vi "Main.vi"(11 "Module Admin":refnum<class "Delacor_lib_QMH_Module Admin.lvclass">) -> ()   [LabVIEW 2020, in "Contabilidad.lvlib"]
doc: "This template is based off of the Queued Message Handler design pattern and the Queued Message Handler project template that ships with LabVIEW.\n\nThe main difference is that the queue is private to this module and communication between modules is performed via Broadcast and Request events.\n\nRequest events are wrapped in public API methods and are handled in the Event Handling Loop (EHL) of this VI. Any module can register for Broadcast events sent by this module. The EHL generates messages based on user interface actions.\n\nThe Message Handling Loop (MHL) processes messages generated by the EHL, or by other messages. The messages are string values, so new messages can be added easily to the Message Cases case structure in the MHL. Each message cluster can also provide an optional value for Message Data, which is a variant that can be converted to whatever message-specific data is required.\n_____\nBased on DQMH Project Template 6.0.0.91."
uses:
  Contabilidad.lvlib
  <vilib>/Delacor/Delacor QMH/Libraries/Module Admin_class/Delacor_lib_QMH_Module Admin.lvclass
  Module Data--cluster.ctl
  Stop Argument--cluster.ctl
  <vilib>/Delacor/Delacor QMH/Libraries/Message Queue_class/Delacor_lib_QMH_Message Queue.lvclass/Delacor_lib_QMH_Message Queue.ctl
  <vilib>/Delacor/Delacor QMH/Libraries/Module Admin_class/Delacor_lib_QMH_Module Admin.lvclass/Delacor_lib_QMH_Module Admin.ctl
  <vilib>/Utility/miscctls.llb/LVPointTypeDef.ctl
  <vilib>/Delacor/Delacor QMH/Libraries/Message Queue_class/Delacor_lib_QMH_Enqueue Message (Single).vi
  <vilib>/Delacor/Delacor QMH/Libraries/Module Admin_class/Delacor_lib_QMH_Get External Launch.vi
  <vilib>/Utility/error.llb/Error Cluster From Error Code.vi
  <vilib>/ErrorRing/Error Ring.xnode
  <vilib>/Delacor/Delacor QMH/Libraries/Message Queue_class/Delacor_lib_QMH_Message Queue.lvclass
  Paquetes Disponibles/Paquetes Disponibles.lvlib
panel:
  out "error out":errorcluster
  out "Status":string
types:
  T1 = typedef "Contabilidad.lvlib/Request Events--cluster.ctl" = cluster{"Stop Module":refnum<user-event>, "Show Panel":refnum<user-event>, "Hide Panel":refnum<user-event>, "Get Module Execution Status":refnum<user-event>, "Show Diagram":refnum<user-event>}
  T2 = typedef "Paquetes Disponibles.lvlib/Broadcast Events--cluster.ctl" = cluster{"Module Did Init":refnum<user-event>, "Status Updated":refnum<user-event>, "Error Reported":refnum<user-event>, "Module Did Stop":refnum<user-event>, "Update Module Execution Status":refnum<user-event>, "Servicio Seleccionado":refnum<user-event>, "Actualizar Credito":refnum<user-event>, "Actualizar Cambio":refnum<user-event>}
  T3 = typedef "Contabilidad.lvlib/Module Data--cluster.ctl" = cluster{"Status":string}
  T4 = enum32{"invalid lock state", "Not Locked", "Locked (No Password)", "Password-protected"}
  T5 = typedef "Contabilidad.lvlib/Stop Argument--cluster.ctl" = cluster{"Origin":string, "Exit via Stop Module Req?":bool, "Wait for Module to stop?":bool}
  T6 = typedef "LVPointTypeDef.ctl" = cluster{"Horizontal":i16, "Vertical":i16}
  T7 = enum32{"Invalid", "Standard", "Closed", "Hidden", "Minimized", "Maximized"}
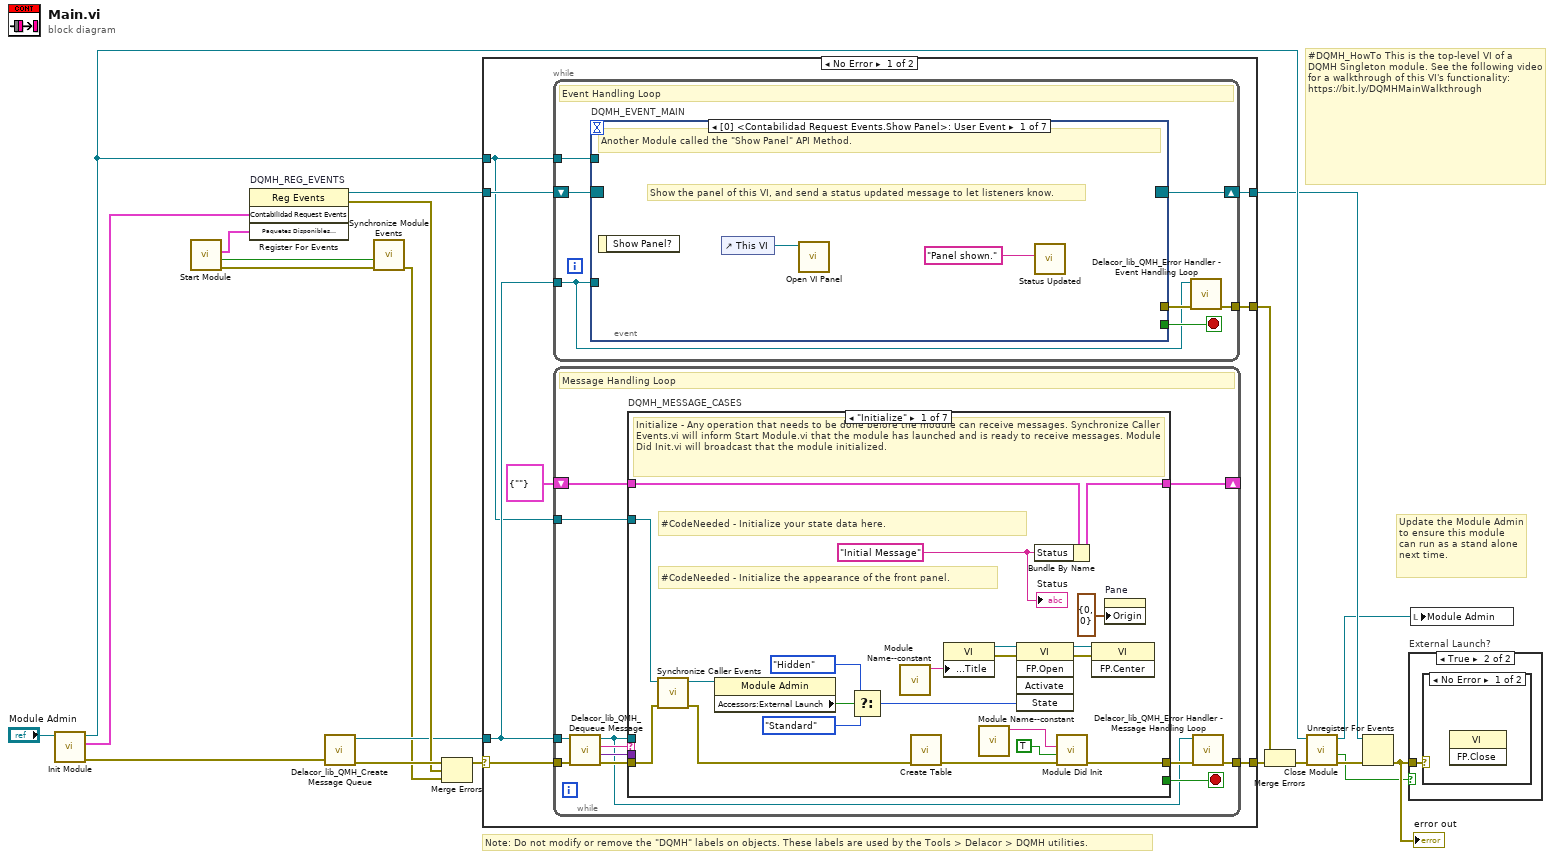
[diagram p0: block diagram]
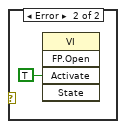
[diagram p3: hidden frame]
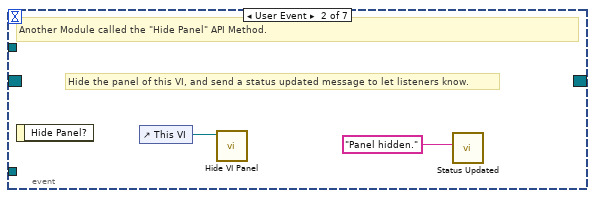
[diagram p4: hidden frame]
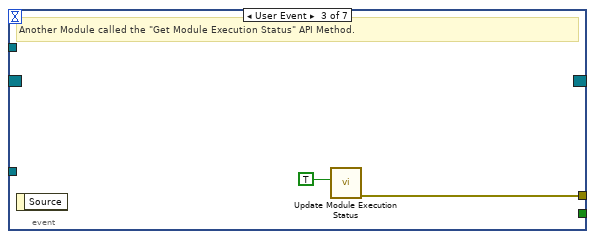
[diagram p5: hidden frame]
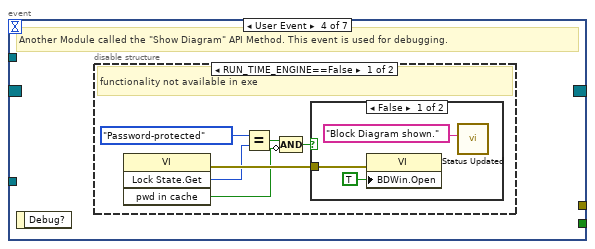
[diagram p6: hidden frame]
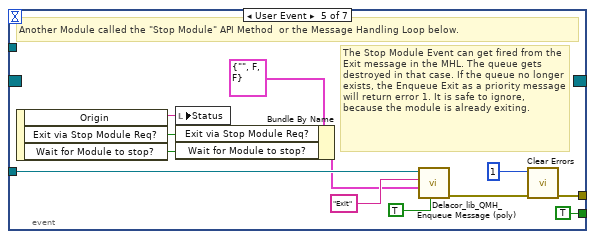
[diagram p9: hidden frame]
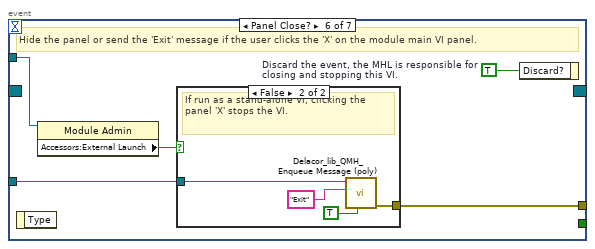
[diagram p10: hidden frame]
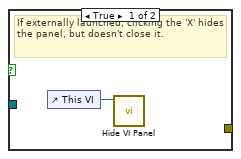
[diagram p11: hidden frame]
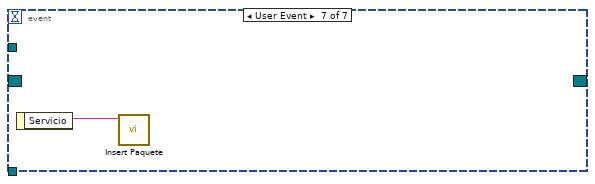
[diagram p12: hidden frame]
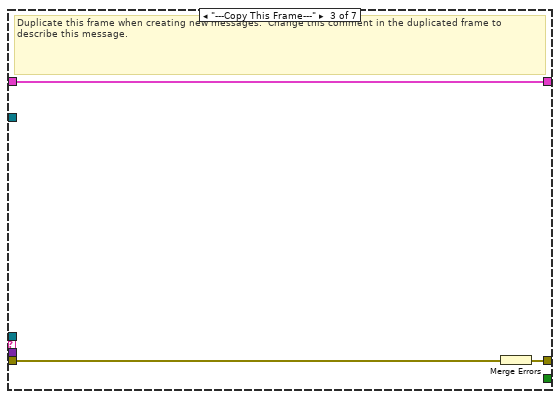
[diagram p14: hidden frame]
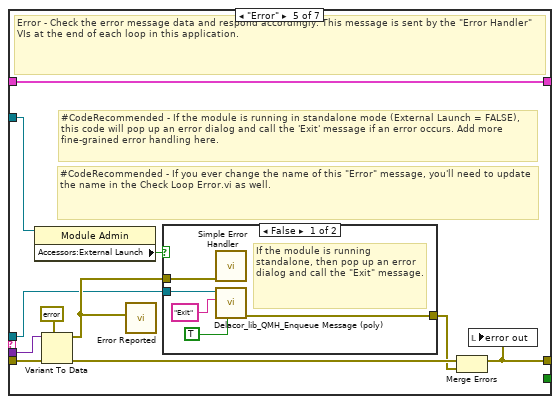
[diagram p16: hidden frame]
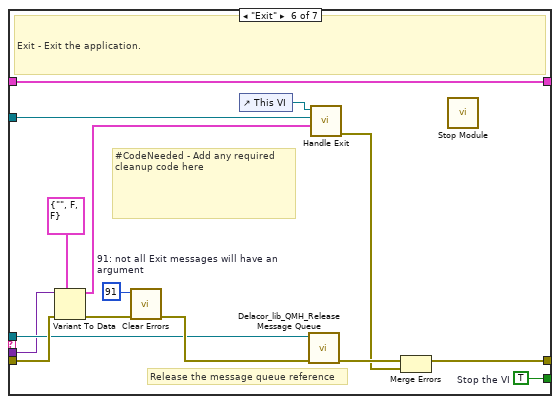
[diagram p18: hidden frame]
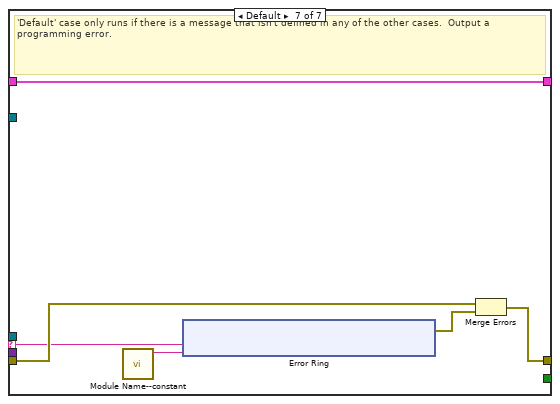
[diagram p19: hidden frame]
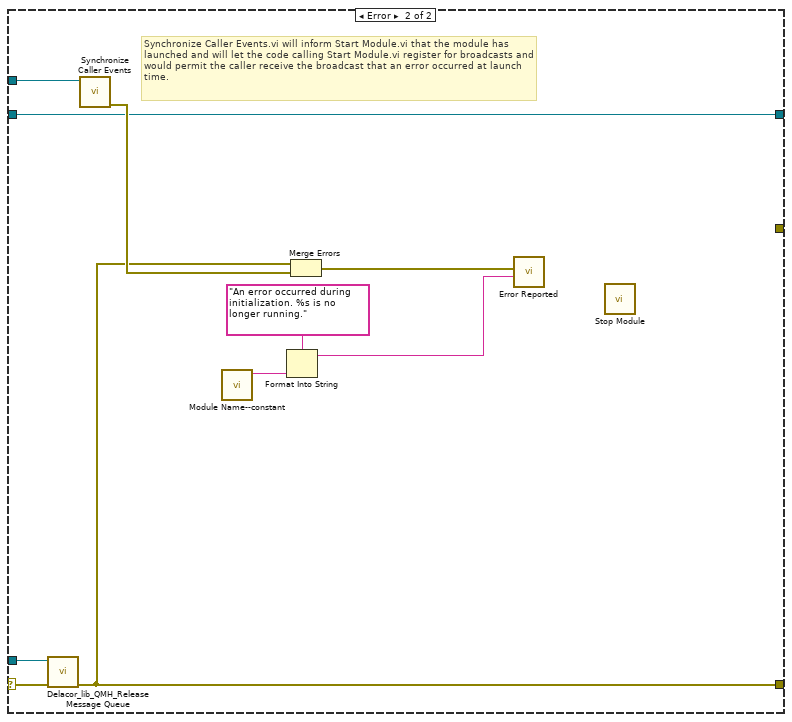
[diagram p20: hidden frame]
diagram:
  # "#DQMH_HowTo This is the top-level VI of a DQMH Singleton module. See the following video for a walkthrough of this VI's functionality: https://bit.ly/DQMHMainWalkthrough"
  # "Note: Do not modify or remove the \"DQMH\" labels on objects. These labels are used by the Tools > Delacor > DQMH utilities."
  # "Update the Module Admin to ensure this module can run as a stand alone next time."
  n1 = call "Init Module.vi"("Singleton Module Admin in"="Module Admin") -> ("error out"=w20:errorcluster, "Contabilidad Request Events"=w9:T1, "Singleton Module Admin out"=w12:refnum<class "Delacor_lib_QMH_Module Admin.lvclass">)  [unwired: 8 in]
  n2 = call "Start Module.vi"() -> ("error out"=w1:errorcluster, "Wait for Event Sync?"=w3:bool, "Paquetes Disponibles Broadcast Events"=w4:T2)  [unwired: 8 in, 1 out]
  n3 = register-events "DQMH_REG_EVENTS"(w9, w4) -> (reference out=w10:refnum<event-registration>, error out=w13:errorcluster)  [unwired: 2 in]
  n4 = call <vilib>:"Delacor_lib_QMH_Create Message Queue.vi"("error in"=w20) -> ("error out"=w15:errorcluster, "Message Queue"=w8:refnum<class "Delacor_lib_QMH_Message Queue.lvclass">)  [unwired: 9 in]
  n5 = call "Synchronize Module Events.vi"("error in"=w1, "Wait for Event Sync?"=w3) -> ("error out"=w2:errorcluster)  [unwired: 9 in]
  n6 = Merge Errors(w15, w13, w2) -> (w14:errorcluster)
  n7 = case shown="No Error" w14 {
    selector: w14 -> [w27 w162]
    tunnel: [w29 w161] -> w21
    tunnel: [w26 w167] -> w11
    tunnel: w10 -> [w24 w167]
    tunnel: w8 -> [w23 w160]
    tunnel: [w28 _] -> w18
    tunnel: w12 -> [w22 w163]
    frame No Error {
      n8 = while {
        tunnel: w23 -> [w30]
        shift-right: [w33] -> w26
        shift-left: w24 -> [w34]
        tunnel: [w35] -> w28
        tunnel: w22 -> [w31]
        stop <- w32 stop-if-true
        # "Event Handling Loop"
        n9 = event "DQMH_EVENT_MAIN" shown="[0] <Contabilidad Request Events.Show Panel>: User Event" {
          selector: w34 -> [_ _ _ _ _ _ _]
          dyn-events: [_ _ _ _ _ _ _] -> w33
          timeout: _ -> [_ _ _ _ _ _ _]
          tunnel: [_ _ _ _ TRUE ("Discard?") _ _] -> w32
          tunnel: w30 -> [_ _ _ _ w59 w66 _]
          tunnel: [_ _ w42 _ w62 w68 _] -> w36
          tunnel: w31 -> [_ _ _ _ _ w65 _]
          event User Event {
            # "Show the panel of this VI, and send a status updated message to let listeners know."
            # "Another Module called the \"Show Panel\" API Method."
            n10 = event-data() -> ()  [unwired: 1 in, 1 out]
            n11 = control-ref of="This VI"() -> (w38:refnum<vi>)
            n12 = call "Open VI Panel.vi"("VI"=w38) -> ()  [unwired: 10 in, 1 out]
            n13 = call "Status Updated.vi"("Status"="Panel shown." ("format string")) -> ()  [unwired: 10 in, 1 out]
          }
          event User Event {
            # "Hide the panel of this VI, and send a status updated message to let listeners know."
            # "Another Module called the \"Hide Panel\" API Method."
            n14 = event-data() -> ()  [unwired: 1 in, 1 out]
            n15 = control-ref of="This VI"() -> (w40:refnum<vi>)
            n16 = call "Hide VI Panel.vi"("VI"=w40) -> ()  [unwired: 10 in, 1 out]
            n17 = call "Status Updated.vi"("Status"="Panel hidden." ("format string")) -> ()  [unwired: 10 in, 1 out]
          }
          event User Event {
            # "Another Module called the \"Get Module Execution Status\" API Method."
            n18 = event-data() -> ()  [unwired: 1 in, 1 out]
            n19 = call "Update Module Execution Status.vi"("Running?"=TRUE) -> ("error out"=w42:errorcluster)  [unwired: 10 in]
          }
          event User Event {
            # "Another Module called the \"Show Diagram\" API Method. This event is used for debugging."
            n20 = event-data() -> ()  [unwired: 1 in, 1 out]
            n21 = disable-structure shown="RUN_TIME_ENGINE==False" {
              frame condition #0 (active) {
                # "functionality not available in exe"
                n22 = invoke class="VI" method="Lock State.Get"() -> (error out=w48:errorcluster, "Get Lock State"=w47:T4, "pwd in cache"=w44:bool)  [unwired: 4 in, 1 out]
                n23 = Equal?(x=T4."Password-protected", y=w47) -> (x = y?=w45:bool)
                n24 = Compound Arithmetic op=AND(w45, invert w44) -> (w43:bool)
                n25 = case shown="False" w43 {
                  tunnel: w48 -> [w51 _]
                  frame False {
                    n26 = property class="VI"(error in=w51, "BDWin.Open"=TRUE ("Block Diagram Window:Open")) -> ()  [unwired: 1 in, 2 out]
                    n27 = call "Status Updated.vi"("Status"="Block Diagram shown." ("format string")) -> ()  [unwired: 10 in, 1 out]
                  }
                  frame True {
                    # "Password-protected VI, and the password is not in the cache. Do not show the diagram."
                  }
                }
              }
              frame condition #1 {
              }
            }
          }
          event User Event {
            # "The Stop Module Event can get fired from the Exit message in the MHL. The queue gets destroyed in that case. If the queue no longer exists, the Enqueue Exit as a priority message will return error 1. It is safe to ignore, because the module is already exiting."
            # "Another Module called the \"Stop Module\" API Method  or the Message Handling Loop below."
            n28 = event-data() -> ("Origin"=w58:string, "Exit via Stop Module Req?"=w54:bool, "Wait for Module to stop?"=w53:bool)  [unwired: 1 in]
            n29 = local write "Status"(w58) -> ()
            n30 = Bundle By Name(cluster=T5 {"Origin"="", "Exit via Stop Module Req?"=FALSE, "Wait for Module to stop?"=FALSE} ("Stop Argument"), "Exit via Stop Module Req?"=w54, "Wait for Module to stop?"=w53) -> (w52:T5)
            n31 = call-poly <vilib>:"Delacor_lib_QMH_Enqueue Message (poly).vi"("Priority Message? (F)"=TRUE, "Message Data"=w52, "Message"="Exit", "Message Queue in"=w59) -> ("error out"=w63:errorcluster)  [unwired: 6 in, 1 out]
            n32 = call <vilib>:"Clear Errors.vi"("error in (no error)"=w63, "specific error code to clear (0: all)"=1) -> ("error out"=w62:errorcluster)  [unwired: 4 in, 1 out]
          }
          event Panel Close? {
            w67 = TRUE  # Discard the event, the MHL is responsible for closing and stopping this VI.
            # "Hide the panel or send the 'Exit' message if the user clicks the 'X' on the module main VI panel."
            n33 = event-data() -> ()  [unwired: 1 in, 1 out]
            n34 = property class="Module Admin"(reference=w65) -> ("Accessors:External Launch"=w64:bool)  [unwired: 1 in, 2 out]
            n35 = case shown="False" w64 {
              tunnel: w66 -> [_ w72]
              tunnel: [_ w73] -> w68
              frame True {
                # "If externally launched, clicking the 'X' hides the panel, but doesn't close it."
                n36 = control-ref of="This VI"() -> (w69:refnum<vi>)
                n37 = call "Hide VI Panel.vi"("VI"=w69) -> ()  [unwired: 10 in, 1 out]
              }
              frame False {
                # "If run as a stand-alone VI, clicking the panel 'X' stops the VI."
                n38 = call-poly <vilib>:"Delacor_lib_QMH_Enqueue Message (poly).vi"("Priority Message? (F)"=TRUE, "Message"="Exit", "Message Queue in"=w72) -> ("error out"=w73:errorcluster)  [unwired: 7 in, 1 out]
              }
            }
            n39 = event-data("Discard?"=w67) -> ()  [unwired: 1 in, 1 out]
          }
          event User Event {
            n40 = event-data() -> ("Servicio"=w74:string)  [unwired: 1 in]
            n41 = call "Insert Paquete.vi"("Paquete"=w74) -> ()  [unwired: 10 in, 1 out]
          }
        }
        n42 = call-dynamic "Delacor_lib_QMH_Error Handler - Event Handling Loop.vi"("error in"=w36, "Message Queue in"=w30) -> ("dup error in"=w35:errorcluster)  [unwired: 8 in, 1 out]
      }
      n43 = while {
        tunnel: w23 -> [w77]
        shift-right: [w81] -> _
        shift-left: T3 {"Status"=""} ("Data Cluster") -> [w82]
        tunnel: w27 -> [w85]
        tunnel: [w83] -> w29
        tunnel: w22 -> [w75]
        stop <- w80 stop-if-true
        # "Message Handling Loop"
        n44 = call-dynamic "Delacor_lib_QMH_Dequeue Message.vi"("error in"=w85, "Message Queue in"=w77) -> ("error out"=w84:errorcluster, "Message Data"=w78:variant, "Message"=w79:string, "Message Queue out"=w76:refnum<class "Delacor_lib_QMH_Message Queue.lvclass">)  [unwired: 6 in]
        n45 = case "DQMH_MESSAGE_CASES" shown="\"Initialize\"" w79 {
          selector: w79 -> [_ _ _ _ _ _ w147]
          tunnel: w76 -> [_ _ _ _ w117 w139 _]
          tunnel: w84 -> [w105 w109 w112 w114 w124 w145 w149]
          tunnel: [w104 w109 w111 w114 w120 w142 w150] -> w86
          tunnel: w82 -> [w95 w108 w110 w113 w119 w138 w148]
          tunnel: [w94 w108 w110 w113 w119 w138 w148] -> w81
          tunnel: [_ _ _ _ _ w137 _] -> w80
          tunnel: w78 -> [_ _ _ _ w118 w136 _]
          tunnel: w75 -> [w96 _ _ _ w116 w131 _]
          frame "Initialize" {
            w90 = "Initial Message" ("Initial Message")
            # "#CodeNeeded - Initialize the appearance of the front panel."
            # "#CodeNeeded - Initialize your state data here."
            # "Initialize - Any operation that needs to be done before the module can receive messages. Synchronize Caller Events.vi will inform Start Module.vi that the module has launched and is ready to receive messages. Module Did Init.vi will broadcast that the module initialized."
            n46 = call "Synchronize Caller Events.vi"("error in (no error)"=w105, "Singleton Module Admin in"=w96) -> ("error out"=w87:errorcluster, "Singleton Module Admin out"=w91:refnum<class "Delacor_lib_QMH_Module Admin.lvclass">)  [unwired: 8 in]
            n47 = property class="Module Admin"(reference=w91) -> ("Accessors:External Launch"=w100:bool)  [unwired: 1 in, 2 out]
            n48 = Select(t=T7."Hidden" ("State"), s=w100, f=T7."Standard" ("State")) -> (s? t:f=w97:T7)
            n49 = call "Module Name--constant.vi"() -> ("Module Name"=w103:string)  [unwired: 11 in]
            n50 = call "Create Table.vi"("error in (no error)"=w87) -> ("error out"=w88:errorcluster)  [unwired: 10 in]
            n51 = property class="VI"("Front Panel.Title"=w103) -> (reference out=w102:refnum<vi>, error out=w107:errorcluster)  [unwired: 2 in]
            n52 = call "Module Name--constant.vi"() -> ("Module Name"=w92:string)  [unwired: 11 in]
            n53 = invoke class="VI" method="FP.Open"(reference=w102, error in=w107, "State"=w97) -> (reference out=w101:refnum<vi>, error out=w106:errorcluster)  [unwired: 2 in, 3 out]
            n54 = Bundle By Name(cluster=w95, "Status"=w90) -> (w94:T3)
            n55 = call "Module Did Init.vi"("error in (no error)"=w88, "Initialized?"=TRUE, "Origin"=w92) -> ("error out"=w104:errorcluster)  [unwired: 8 in]
            n56 = invoke class="VI" method="FP.Center"(reference=w101, error in=w106) -> ()  [unwired: 1 in, 3 out]
            n57 = property on="Pane" class="Pane"("Origin"=T6 {"Horizontal"=0, "Vertical"=0}) -> ()  [unwired: 2 in, 2 out]
            "Status" <- w90
          }
          frame "---Module Specific---" {
            # "Separator -- The following cases handle messages specific to this Module."
          }
          frame "---Copy This Frame---" {
            # "Duplicate this frame when creating new messages.  Change this comment in the duplicated frame to describe this message."
            n58 = Merge Errors(w112) -> (w111:errorcluster)
          }
          frame "---Exit and Error Handling---" {
            # "Separator - The following cases handle errors and exit messages."
          }
          frame "Error" {
            # "#CodeRecommended - If you ever change the name of this \"Error\" message, you'll need to update the name in the Check Loop Error.vi as well."
            # "#CodeRecommended - If the module is running in standalone mode (External Launch = FALSE), this code will pop up an error dialog and call the 'Exit' message if an error occurs. Add more fine-grained error handling here."
            # "Error - Check the error message data and respond accordingly. This message is sent by the \"Error Handler\" VIs at the end of each loop in this application."
            n59 = property class="Module Admin"(reference=w116) -> ("Accessors:External Launch"=w115:bool)  [unwired: 1 in, 2 out]
            n60 = Variant To Data(error in=w124, type=errorcluster {"status"=FALSE, "code"=0, "source"=""} ("error constant"), Variant=w118) -> (data=w125:errorcluster, error out=w122:errorcluster)
            n61 = call "Error Reported.vi"("Error"=w125) -> ()  [unwired: 10 in, 1 out]
            n62 = case shown="False" w115 {
              tunnel: [w130 _] -> w121
              tunnel: w117 -> [w128 _]
              tunnel: w125 -> [w129 _]
              frame False {
                # "If the module is running standalone, then pop up an error dialog and call the \"Exit\" message."
                n63 = call <vilib>:"Simple Error Handler.vi"("error in (no error)"=w129) -> ()  [unwired: 4 in, 5 out]
                n64 = call-poly <vilib>:"Delacor_lib_QMH_Enqueue Message (poly).vi"("Priority Message? (F)"=TRUE, "Message"="Exit", "Message Queue in"=w128) -> ("error out"=w130:errorcluster)  [unwired: 7 in, 1 out]
              }
              frame True {
                # "If the module was launched externally, calling the Error Reported broadcast VI is the only action performed by the \"Error\" message. The module's caller can then process the error appropriately."
              }
            }
            n65 = Merge Errors(w122, w121) -> (w120:errorcluster)
            n66 = local write "error out"(w120) -> ()
          }
          frame "Exit" {
            w135 = 91  # 91: not all Exit messages will have an argument
            w137 = TRUE  # Stop the VI
            # "Release the message queue reference"
            # "#CodeNeeded - Add any required cleanup code here"
            # "Exit - Exit the application."
            n67 = Variant To Data(error in=w145, type=T5 {"Origin"="", "Exit via Stop Module Req?"=FALSE, "Wait for Module to stop?"=FALSE} ("Stop Argument"), Variant=w136) -> (data=w133:T5, error out=w141:errorcluster)
            n68 = call <vilib>:"Clear Errors.vi"("error in (no error)"=w141, "specific error code to clear (0: all)"=w135) -> ("error out"=w144:errorcluster)  [unwired: 4 in, 1 out]
            n69 = control-ref of="This VI"() -> (w132:refnum<vi>)
            n70 = call-dynamic "Delacor_lib_QMH_Release Message Queue.vi"("error in"=w144, "Message Queue"=w139) -> ("error out"=w143:errorcluster)  [unwired: 9 in]
            n71 = call "Handle Exit.vi"("Stop Argument"=w133, "Admin in"=w131, "VI reference"=w132) -> ("error out"=w140:errorcluster)  [unwired: 7 in, 1 out]
            n72 = Merge Errors(w143, w140) -> (w142:errorcluster)
            n73 = call "Stop Module.vi"() -> ()  [unwired: 11 in, 1 out]
          }
          frame Default {
            # "'Default' case only runs if there is a message that isn't defined in any of the other cases.  Output a programming error."
            n74 = call "Module Name--constant.vi"() -> ("Module Name"=w146:string)  [unwired: 11 in]
            n75 = xnode "Error Ring"("parameter 0"=w147, "parameter 1"=w146) -> ("error out"=w151:errorcluster)
            n76 = Merge Errors(w149, w151) -> (w150:errorcluster)
          }
        }
        n77 = call-dynamic "Delacor_lib_QMH_Error Handler - Message Handling Loop.vi"("error in"=w86, "Message Queue in"=w76) -> ("dup error in"=w83:errorcluster)  [unwired: 8 in, 1 out]
      }
    }
    frame Error {
      # "Synchronize Caller Events.vi will inform Start Module.vi that the module has launched and will let the code calling Start Module.vi register for broadcasts and would permit the caller receive the broadcast that an error occurred at launch time."
      n78 = call-dynamic "Delacor_lib_QMH_Release Message Queue.vi"("error in"=w162, "Message Queue"=w160) -> ("error out"=w161:errorcluster)  [unwired: 9 in]
      n79 = call "Synchronize Caller Events.vi"("Singleton Module Admin in"=w163) -> ("error out"=w168:errorcluster)  [unwired: 9 in, 1 out]
      n80 = call "Module Name--constant.vi"() -> ("Module Name"=w166:string)  [unwired: 11 in]
      n81 = Format Into String(format string="An error occurred during initialization. %s is no longer running.", w166) -> (resulting string=w164:string)  [unwired: 2 in, 1 out]
      n82 = Merge Errors(w161, w168) -> (w169:errorcluster)
      n83 = call "Error Reported.vi"("Additional Information"=w164, "Error"=w169) -> ()  [unwired: 9 in, 1 out]
      n84 = call "Stop Module.vi"() -> ()  [unwired: 11 in, 1 out]
    }
  }
  n85 = Merge Errors(w18, w21) -> (w17:errorcluster)
  n86 = call "Close Module.vi"("error in (no error)"=w17, "Module Admin in"=w12) -> ("error out"=w19:errorcluster, "External Launch"=w5:bool, "Module Admin out"=w6:refnum<class "Delacor_lib_QMH_Module Admin.lvclass">)  [unwired: 7 in]
  n87 = Unregister For Events(event registration refnum=w11, error in=w19) -> (error out=w16:errorcluster)
  "error out" <- w16
  n88 = case "External Launch?" shown="True" w5 {
    tunnel: w16 -> [_ w170]
    frame False {
    }
    frame True {
      n89 = case shown="No Error" w170 {
        frame No Error {
          n90 = invoke class="VI" method="FP.Close"() -> ()  [unwired: 3 in, 3 out]
        }
        frame Error {
          n91 = invoke class="VI" method="FP.Open"("Activate"=TRUE ("Activate?")) -> ()  [unwired: 4 in, 5 out]
        }
      }
    }
  }
  n92 = local write "Module Admin"(w6) -> ()
